vi "WPI_AccelerometerInternalGetAcceleration.vi"(8 "error in":errorcluster, 11 "AccelerometerDevRef":T1={"DevStatus"={"status"=FALSE, "code"=0, "source"=""}, "Scaling"={"Gain (VoltsPerG)"=0.0, "Center Voltage"=0.0}, "Analog Channels"={"X-Axis"=enum."Invalid", "Y-Axis"=enum."Invalid", "Z-Axis"=enum."Invalid"}, "I2C Bus"=enum."Invalid", "SPI Bus"=enum."Invalid", "Accel Range"=0, "ADXL Axes"={"X-Axis"=FALSE, "Y-Axis"=FALSE, "Z-Axis"=FALSE}, "Handle"=0, "Device Address"=0, "Accel Type"=enum."Analog"} {"Device Address" format="%.0x"; "Accel Range" items=["+/- 2 g", "+/- 4 g", "+/- 8 g", "+/- 16 g"]}) -> (0 "error out":errorcluster, 2 "Accelerations":T9, 3 "AccelerometerDevRef":T1={"DevStatus"={"status"=FALSE, "code"=0, "source"=""}, "Scaling"={"Gain (VoltsPerG)"=0.0, "Center Voltage"=0.0}, "Analog Channels"={"X-Axis"=enum."Invalid", "Y-Axis"=enum."Invalid", "Z-Axis"=enum."Invalid"}, "I2C Bus"=enum."Invalid", "SPI Bus"=enum."Invalid", "Accel Range"=0, "ADXL Axes"={"X-Axis"=FALSE, "Y-Axis"=FALSE, "Z-Axis"=FALSE}, "Handle"=0, "Device Address"=0, "Accel Type"=enum."Analog"} {"Device Address" format="%.0x"; "Accel Range" items=["+/- 2 g", "+/- 4 g", "+/- 8 g", "+/- 16 g"]})   [LabVIEW 2017]
uses:
  <vilib>/Rock Robotics/WPI/Accelerometer/WPI_AccelerometerDevRef.ctl
  <vilib>/Rock Robotics/WPI/Accelerometer/WPI_AccelerometerScaling.ctl
  <vilib>/Rock Robotics/WPI/Accelerometer/WPI_AccelerometerAnalogChannels.ctl
  <vilib>/Rock Robotics/SystemInterfaces/AI/FPGA_AIChannel.ctl
  <vilib>/Rock Robotics/SystemInterfaces/i2clib/i2c_bus.ctl
  <vilib>/Rock Robotics/SystemInterfaces/spilib/spi_bus.ctl
  <vilib>/Rock Robotics/WPI/Accelerometer/ADXL345 Range.ctl
  <vilib>/Rock Robotics/WPI/Accelerometer/WPI_AccelerometerADXL345 Axes.ctl
  <vilib>/Rock Robotics/WPI/Accelerometer/InternalAccelerometer/WPI_Accelerometer_Internal_MMA8452Q_Registers.ctl
panel:
  # "ADXL"
  # "Analog"
  # "ADXL"
  # "Analog"
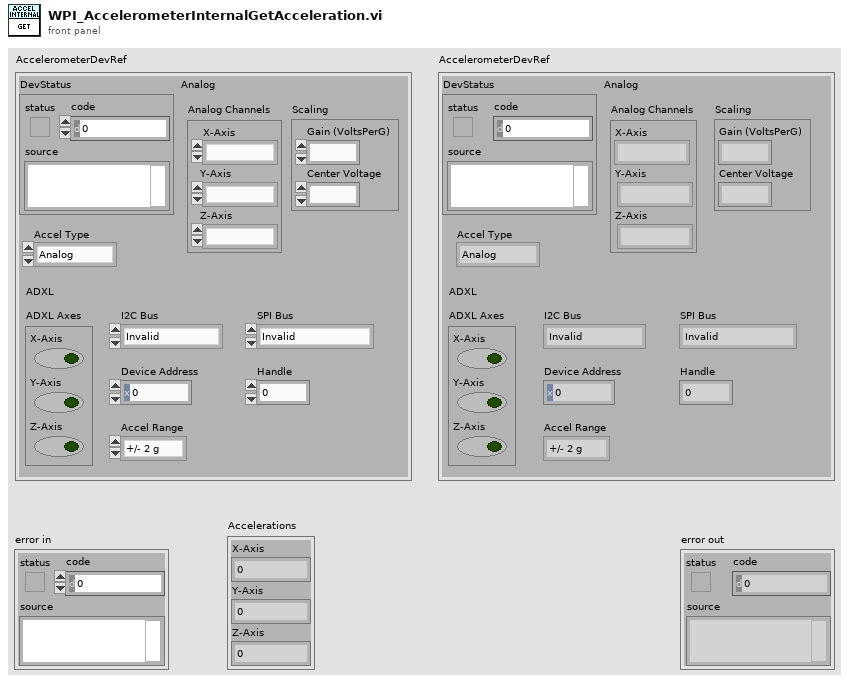
[diagram p1: front panel]
types:
  T1 = typedef "WPI_AccelerometerDevRef.ctl" = cluster{"DevStatus":errorcluster, "Scaling":T2, "Analog Channels":T3, "I2C Bus":T5, "SPI Bus":T6, "Accel Range":T7, "ADXL Axes":T8, "Handle":i32, "Device Address":u8, "Accel Type":enum16{"Analog", "ADXL345 I2C", "ADXL345 SPI", "Internal", "ADXL362 SPI"}}
  T2 = typedef "WPI_AccelerometerScaling.ctl" = cluster{"Gain (VoltsPerG)":dbl, "Center Voltage":dbl}
  T3 = typedef "WPI_AccelerometerAnalogChannels.ctl" = cluster{"X-Axis":T4, "Y-Axis":T4, "Z-Axis":T4}
  T4 = typedef "FPGA_AIChannel.ctl" = enum8{"AI 0", "AI 1", "AI 2", "AI 3", "AI MXP 0", "AI MXP 1", "AI MXP 2", "AI MXP 3", "Invalid"}
  T5 = typedef "i2c_bus.ctl" = enum16{"I2C On-Board", "I2C MXP", "Invalid"}
  T6 = typedef "spi_bus.ctl" = enum16{"SPI On-Board, CS0", "SPI On-Board, CS1", "SPI On-Board, CS2", "SPI On-Board, CS3", "SPI MXP", "Invalid"}
  T7 = typedef "ADXL345 Range.ctl" = u8
  T8 = typedef "WPI_AccelerometerADXL345 Axes.ctl" = cluster{"X-Axis":bool, "Y-Axis":bool, "Z-Axis":bool}
  T9 = cluster{"X-Axis":dbl, "Y-Axis":dbl, "Z-Axis":dbl}
  T10 = typedef "WPI_Accelerometer_Internal_MMA8452Q_Registers.ctl" = u8
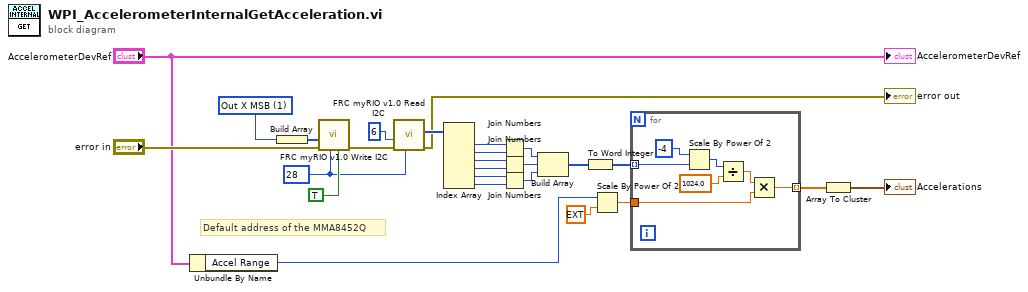
[diagram p0: block diagram]
diagram:
  w2 = T10 1 items=["Status"=0, "Out X MSB"=1, "Out X LSB"=2, "Out Y MSB"=3, "Out Y LSB"=4, "Out Z MSB"=5, "Out Z LSB"=6, "Who Am I"=13, "XYZ Data Config"=14, "Ctrl Reg 1"=42]
  w21 = u8 28 ("Accel.ADDR")
  # "Default address of the MMA8452Q"
  n1 = Unbundle By Name("AccelerometerDevRef") -> ("Accel Range"=w3:T7)
  n2 = Build Array(w2) -> (w26:T10[])
  n3 = call <vilib>:"FRC myRIO v1.0 Write I2C.vi"("Keep Bus Busy"=TRUE, "Slave Address (7-bit)"=w21, "Error In (No Error)"="error in", "Data to Write"=w26) -> ("error out"=w24:errorcluster)  [unwired: 7 in]
  n4 = call <vilib>:"FRC myRIO v1.0 Read I2C.vi"("Slave Address (7-bit)"=w21, "Error In (No Error)"=w24, "Bytes to Read"=u32 6) -> ("error out"=→"error out":errorcluster, "Data Read"=w22:u8[])  [unwired: 7 in]
  n5 = Index Array(array=w22) -> (element #1=w19:u8, element #2=w18:u8, element #3=w17:u8, element #4=w16:u8, element #5=w14:u8, element #6=w15:u8)  [unwired: 6 in]
  n6 = Join Numbers(hi=w19, lo=w18) -> ((hi.lo)=w13:u16)
  n7 = Join Numbers(hi=w17, lo=w16) -> ((hi.lo)=w12:u16)
  n8 = Join Numbers(hi=w14, lo=w15) -> ((hi.lo)=w11:u16)
  n9 = Build Array(w13, w12, w11) -> (w10:u16[])
  n10 = To Word Integer(number=w10) -> (16bit integer=w8:i16[])
  n11 = Scale By Power Of 2(n=w3, x=ext 1.0) -> (x*2^n=w6:ext)
  n12 = for {
    tunnel: w8 -> [w33] mode=indexing
    tunnel: w6 -> [w27]
    tunnel: [w31] -> w9 mode=indexing
    n13 = Scale By Power Of 2(n=i16 -4, x=w33) -> (x*2^n=w29:i16)
    n14 = Divide(x=w29, y=1024.0) -> (x/y=w28:dbl)
    n15 = Multiply(x=w28, y=w27) -> (x*y=w31:ext)
  }
  n16 = Array To Cluster(array=w9) -> (cluster=→"Accelerations":cluster{"[0]":ext, "[1]":ext, "[2]":ext})
  "AccelerometerDevRef" <- "AccelerometerDevRef"
